vi "調整Label位置.vi"   [LabVIEW 2015]
types:
  T1 = typedef "LVPositionTypeDef.ctl" = cluster{"Left":i32, "Top":i32}
  T2 = typedef "LVRectTypeDef.ctl" = cluster{"Left":i16, "Top":i16, "Right":i16, "Bottom":i16}
  T3 = typedef "LVBoundsTypeDef.ctl" = cluster{"Width":u32, "Height":u32}
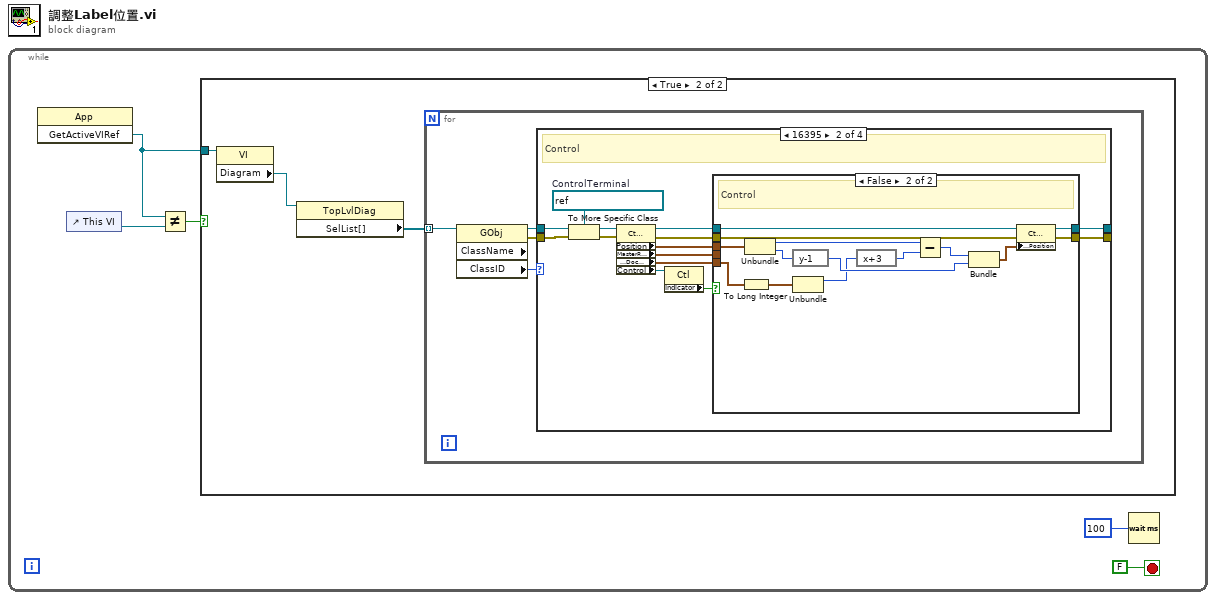
[diagram p0: block diagram]
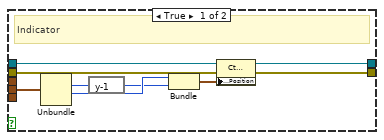
[diagram p4: hidden frame]
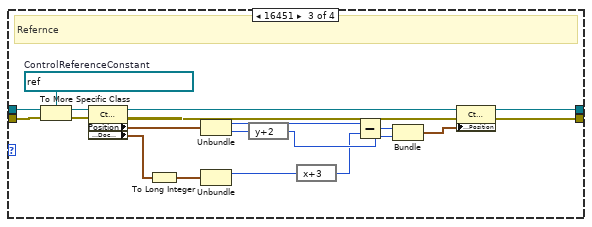
[diagram p5: hidden frame]
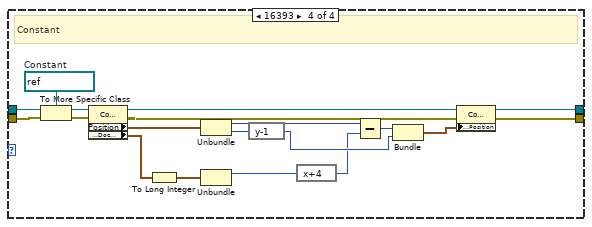
[diagram p6: hidden frame]
diagram:
  n1 = while {
    stop <- FALSE stop-if-true
    n2 = invoke class="App" method="GetActiveVIRef"() -> ("GetActiveVIRef"=w4:refnum<vi>)  [unwired: 3 in, 2 out]
    n3 = control-ref of="This VI"() -> (w5:refnum<vi>)
    n4 = Not Equal?(x=w4, y=w5) -> (x != y?=w3:bool)
    n5 = case shown="True" w3 {
      tunnel: w4 -> [_ w6]
      frame False {
      }
      frame True {
        n6 = property class="VI"(reference=w6) -> ("Diagram"=w8:refnum<vi>)  [unwired: 1 in, 2 out]
        n7 = property class="TopLvlDiag"(reference=w8) -> ("SelList[]"=w7:refnum<vi>[])  [unwired: 1 in, 2 out]
        n8 = for {
          tunnel: w7 -> [w10] mode=indexing
          n9 = property on="Property Node" class="GObj" props=["ClassName", "ClassID"](reference=w10) -> (reference out=w9:refnum<vi>, error out=w11:errorcluster, "ClassID"=w12:u32)  [unwired: 1 in, 1 out]
          n10 = case shown="16395" w12 {
            tunnel: w11 -> [w13 w26 w70 w73]
            tunnel: w9 -> [w14 w27 w69 w74]
            tunnel: [w14 w25 w68 w72] -> _
            tunnel: [w13 w24 w67 w71] -> _
            frame Default {
            }
            frame 16395 {
              w28 = refnum<vi> refnum  # ControlTerminal
              # "Control"
              n11 = To More Specific Class(target class=w28, reference=w27, error in=w26) -> (specific class reference=w22:refnum<vi>, error out=w16:errorcluster)
              n12 = property on="Property Node" class="CtrlTerm"(reference=w22, error in=w16) -> (reference out=w23:refnum<vi>, error out=w15:errorcluster, "Position"=w21:T1, "MasterRect"=w18:T2, "Label.Doc Bounds"=w19:T3, "Control"=w17:refnum<vi>)
              n13 = property on="Property Node" class="Ctl"(reference=w17) -> ("Indicator"=w20:bool)  [unwired: 1 in, 2 out]
              n14 = case shown="False" w20 {
                tunnel: [w35 w43] -> w25
                tunnel: [w34 w42] -> w24
                tunnel: w15 -> [w36 w40]
                tunnel: w23 -> [w33 w41]
                tunnel: w21 -> [_ w39]
                tunnel: w19 -> [_ w38]
                tunnel: w18 -> [w31 _]
                frame True {
                  # "Indicator"
                  n15 = Unbundle(w31) -> ("Top"=w30:i16, "Right"=w32:i16)  [unwired: 2 out]
                  n16 = expression code="y-1"(w30) -> (w29:i16)
                  n17 = Bundle("Right"=w32, "Top"=w29) -> (w37:cluster{"Right":i16, "Top":i16})  [unwired: 1 in]
                  n18 = property on="Property Node" class="CtrlTerm"(reference=w33, error in=w36, "Label.Position"=w37) -> (reference out=w35:refnum<vi>, error out=w34:errorcluster)
                }
                frame False {
                  # "Control"
                  n19 = To Long Integer(number=w38) -> (32bit integer=w44:cluster{"Width":i32, "Height":i32})
                  n20 = Unbundle(w39) -> ("Left"=w47:i32, "Top"=w49:i32)
                  n21 = expression code="y-1"(w49) -> (w50:i32)
                  n22 = Unbundle(w44) -> ("Width"=w48:i32)  [unwired: 1 out]
                  n23 = expression code="x+3"(w48) -> (w46:i32)
                  n24 = Subtract(x=w47, y=w46) -> (x-y=w45:i32)
                  n25 = Bundle(w45, "Top"=w50) -> (w51:cluster{i32, "Top":i32})  [unwired: 1 in]
                  n26 = property on="Property Node" class="CtrlTerm"(reference=w41, error in=w40, "Label.Position"=w51) -> (reference out=w43:refnum<vi>, error out=w42:errorcluster)
                }
              }
            }
            frame 16451 {
              w66 = refnum<vi> refnum  # ControlReferenceConstant
              # "Refernce"
              n27 = To More Specific Class(target class=w66, reference=w69, error in=w70) -> (specific class reference=w65:refnum<vi>, error out=w64:errorcluster)
              n28 = property on="Property Node" class="CtrlRefConst"(reference=w65, error in=w64) -> (reference out=w63:refnum<vi>, error out=w54:errorcluster, "Position"=w62:T1, "Label.Doc Bounds"=w53:T3)
              n29 = To Long Integer(number=w53) -> (32bit integer=w52:cluster{"Width":i32, "Height":i32})
              n30 = Unbundle(w62) -> ("Left"=w57:i32, "Top"=w59:i32)
              n31 = Unbundle(w52) -> ("Width"=w58:i32)  [unwired: 1 out]
              n32 = expression code="y+2"(w59) -> (w60:i32)
              n33 = expression code="x+3"(w58) -> (w56:i32)
              n34 = Subtract(x=w57, y=w56) -> (x-y=w55:i32)
              n35 = Bundle(w55, "Top"=w60) -> (w61:cluster{i32, "Top":i32})  [unwired: 1 in]
              n36 = property on="Property Node" class="CtrlRefConst"(reference=w63, error in=w54, "Label.Position"=w61) -> (reference out=w68:refnum<vi>, error out=w67:errorcluster)
            }
            frame 16393 {
              w89 = refnum<vi> refnum  # Constant
              # "Constant"
              n37 = To More Specific Class(target class=w89, reference=w74, error in=w73) -> (specific class reference=w88:refnum<vi>, error out=w87:errorcluster)
              n38 = property on="Property Node" class="Const"(reference=w88, error in=w87) -> (reference out=w86:refnum<vi>, error out=w77:errorcluster, "Position"=w85:T1, "Label.Doc Bounds"=w76:T3)
              n39 = To Long Integer(number=w76) -> (32bit integer=w75:cluster{"Width":i32, "Height":i32})
              n40 = Unbundle(w85) -> ("Left"=w80:i32, "Top"=w82:i32)
              n41 = Unbundle(w75) -> ("Width"=w81:i32)  [unwired: 1 out]
              n42 = expression code="y-1"(w82) -> (w83:i32)
              n43 = expression code="x+4"(w81) -> (w79:i32)
              n44 = Subtract(x=w80, y=w79) -> (x-y=w78:i32)
              n45 = Bundle(w78, "Top"=w83) -> (w84:cluster{i32, "Top":i32})  [unwired: 1 in]
              n46 = property on="Property Node" class="Const"(reference=w86, error in=w77, "Label.Position"=w84) -> (reference out=w72:refnum<vi>, error out=w71:errorcluster)
            }
          }
        }
      }
    }
    n47 = Wait (ms)(milliseconds to wait=u32 100) -> ()  [unwired: 1 out]
  }
